vi "test_default_value.vi"() -> ()   [LabVIEW 2021]
uses:
  Child/Child.lvclass
panel:
  out "message 2":string
  out "message":string
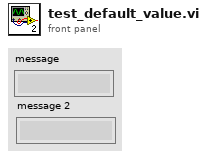
[diagram p1: front panel]
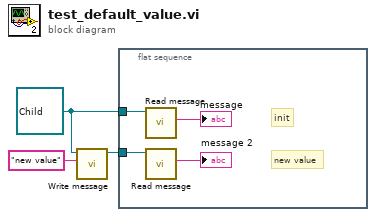
[diagram p0: block diagram]
diagram:
  w3 = refnum<class "Child.lvclass"> refnum ("Child.lvclass")
  n1 = call-dynamic "Write message.vi"("message"="new value", "Child in"=w3) -> ("Child out"=w2:refnum<class "Child.lvclass">)  [unwired: 8 in, 1 out]
  n2 = flat-sequence {
    tunnel: w3 -> [w7]
    tunnel: w2 -> [w4]
    frame #0 {
      # "new value"
      # "init"
      n3 = call-dynamic "Read message.vi"("Child in"=w7) -> ("message"=→"message":string)  [unwired: 8 in, 2 out]
      n4 = call-dynamic "Read message.vi"("Child in"=w4) -> ("message"=→"message 2":string)  [unwired: 8 in, 2 out]
    }
  }
